vi "TurnToAngle.vi"(6 "Setpoint":dbl, 7 "output range":cluster{"output high":dbl, "output low":dbl}, 8 "error in (no error)":errorcluster, 9 "Z Drive PID Gains":T1, 10 "GyroDevRef":T2 {"Sample Rate" min=0.25 max=100.0 step=0.25}, 11 "Setpoint 2":dbl) -> (0 "error out":errorcluster, 3 "Boolean":bool)   [LabVIEW 2016]
uses:
  <vilib>/Rock Robotics/WPI/Gyro/WPI_GyroDevRef.ctl
  <vilib>/Rock Robotics/SystemInterfaces/AI/FPGA_AIChannel.ctl
  <vilib>/Rock Robotics/SystemInterfaces/spilib/spi_bus.ctl
  <vilib>/addons/control/pid/pid.llb/PID (DBL).vi
  <vilib>/addons/control/pid/NI_PID_pid.lvlib
panel:
  # "Analog"
  # "XRS"
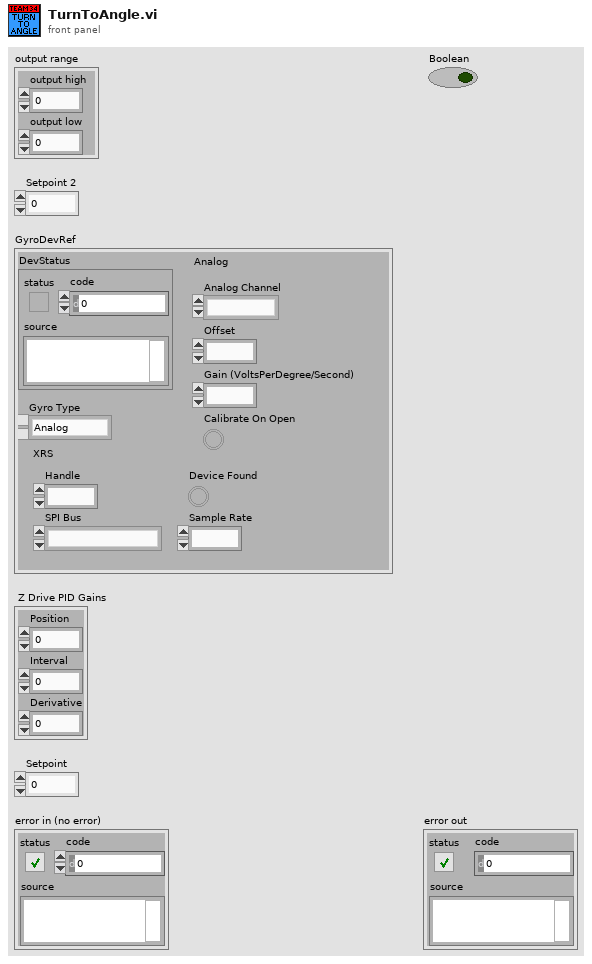
[diagram p1: front panel]
types:
  T1 = cluster{"Position":dbl, "Interval":dbl, "Derivative":dbl}
  T2 = typedef "WPI_GyroDevRef.ctl" = cluster{"DevStatus":errorcluster, "Analog Channel":T3, "Offset":dbl, "Gain (VoltsPerDegree/Second)":dbl, "Gyro Type":enum16{"Analog", "XRS450"}, "Handle":i32, "SPI Bus":T4, "Device Found":bool, "Sample Rate":dbl, "Calibrate On Open":bool}
  T3 = typedef "FPGA_AIChannel.ctl" = enum8{"AI 0", "AI 1", "AI 2", "AI 3", "AI MXP 0", "AI MXP 1", "AI MXP 2", "AI MXP 3", "Invalid"}
  T4 = typedef "spi_bus.ctl" = enum16{"SPI On-Board, CS0", "SPI On-Board, CS1", "SPI On-Board, CS2", "SPI On-Board, CS3", "SPI MXP", "Invalid"}
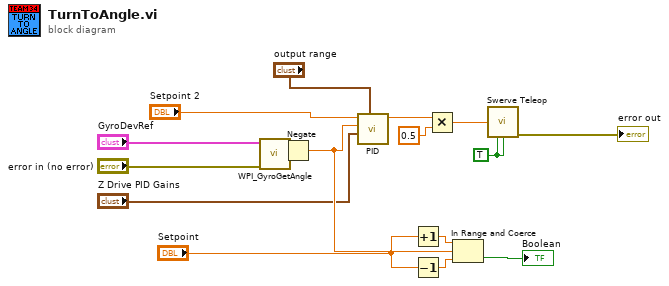
[diagram p0: block diagram]
diagram:
  w6 = TRUE ("Robot Centric?")
  n1 = call <vilib>:"WPI_GyroGetAngle.vi"("error in"="error in (no error)", "GyroDevRef"="GyroDevRef") -> ("Angle"=w15:dbl)  [unwired: 5 in, 4 out]
  n2 = Negate(x=w15) -> (-x=w16:dbl)
  n3 = call-poly <vilib>:"PID.vi"("output range"="output range", "PID gains"="Z Drive PID Gains", "process variable"=w16, "setpoint"="Setpoint 2") -> ("output"=w3:dbl)  [unwired: 6 in, 1 out]
  n4 = Increment(x="Setpoint") -> (x+1=w9:dbl)
  n5 = Decrement(x="Setpoint") -> (x-1=w10:dbl)
  n6 = Multiply(x=w3, y=0.5) -> (x*y=w14:dbl)
  n7 = In Range and Coerce(upper limit=w9, x=w16, lower limit=w10) -> (In Range?=→"Boolean":bool)  [unwired: 1 out]
  n8 = call "Swerve Teleop.vi"("Z"=w14, "Robot Centric?"=w6, "Autonomous?"=w6) -> ("Error Out"=→"error out":errorcluster)  [unwired: 8 in, 4 out]
